vi "Execute.vi"(8 "error in (no error)":errorcluster, 10 "System In":refnum<class "abs_System.lvclass">, 11 "Node in":refnum<class "Parallel_Interleaved.lvclass">) -> (0 "error out":errorcluster, 1 "Status":T1, 2 "System Out":refnum<class "abs_System.lvclass">, 3 "Node out":refnum<class "Parallel_Interleaved.lvclass">)   [LabVIEW 2021, in "BT.lvlib" / "Parallel_Interleaved.lvclass"]
uses:
  Parallel_Interleaved/Parallel_Interleaved.lvclass
  C:/Users/Tim/Documents/GitHub/LV_Behaviour_Tree/Source/Support/abs_Composite/abs_Composite.lvclass
  C:/Users/Tim/Documents/GitHub/LV_Behaviour_Tree/Source/Support/abs_Parallel/abs_Parallel.lvclass
  abs_Node/Status.ctl
  abs_System/abs_System.lvclass
  Parallel_Interleaved/Parallel_Interleaved.lvclass/Parallel_Interleaved.ctl
  abs_Composite/abs_Composite.lvclass/abs_Composite.ctl
  abs_Composite/Properties/Read Index.vi
  abs_Composite/Properties/Read Num Nodes.vi
  abs_Composite/Properties/Write Index.vi
  Parallel_Interleaved/Properties/Read Always Repeat First Node.vi
  abs_Parallel.lvclass
  abs_Node/abs_Node.lvclass
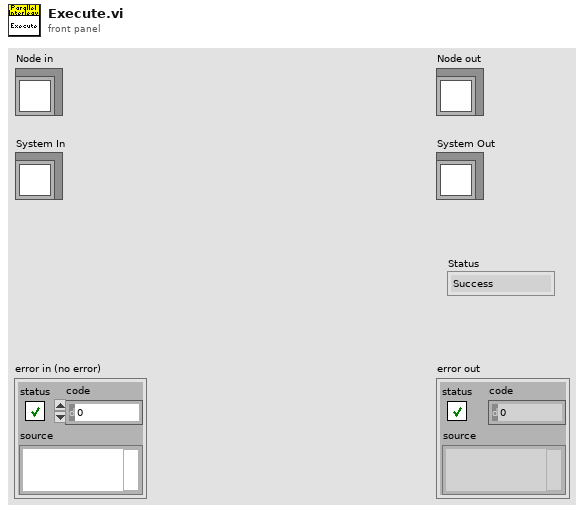
[diagram p1: front panel]
types:
  T1 = typedef "BT.lvlib/abs_Node.lvclass/Status.ctl" = enum16{"Success", "Failure", "Running"}
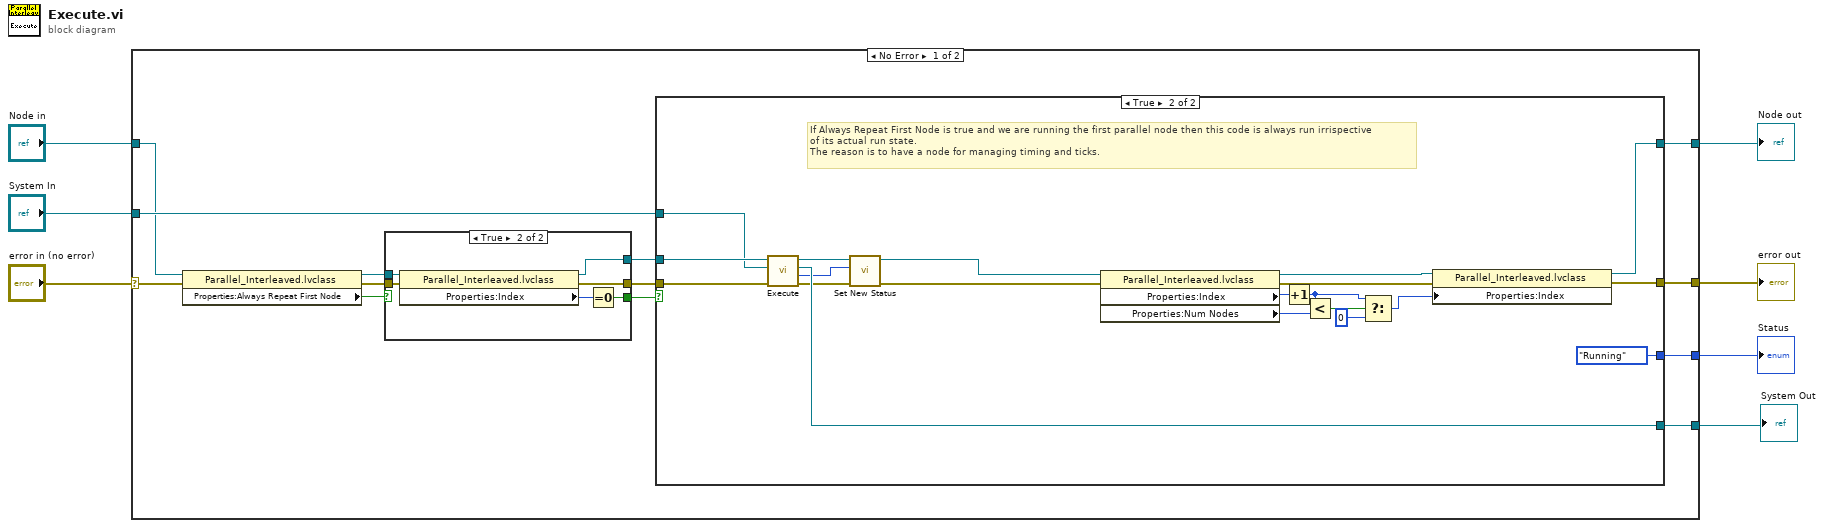
[diagram p0: block diagram]
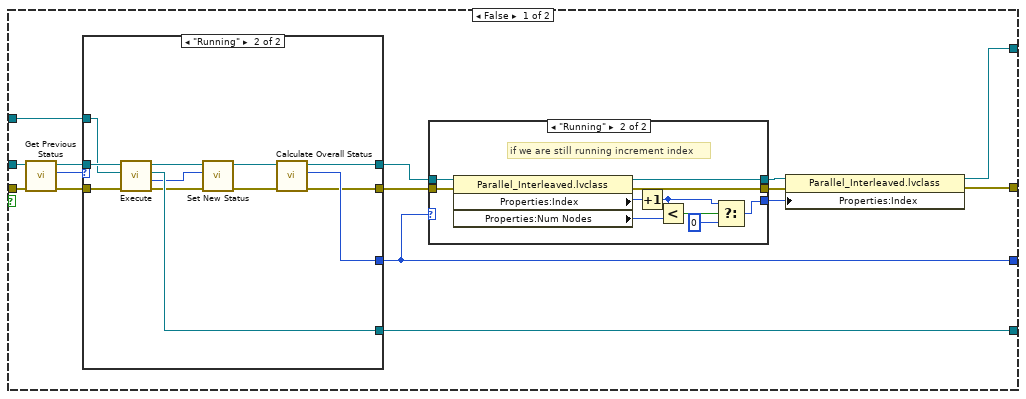
[diagram p2: hidden frame]
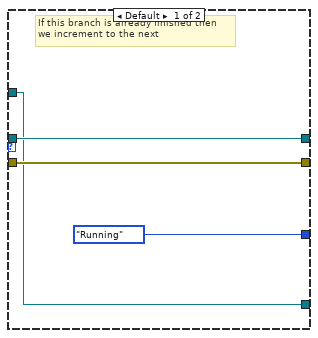
[diagram p3: hidden frame]
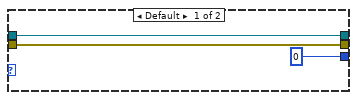
[diagram p4: hidden frame]
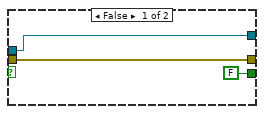
[diagram p5: hidden frame]
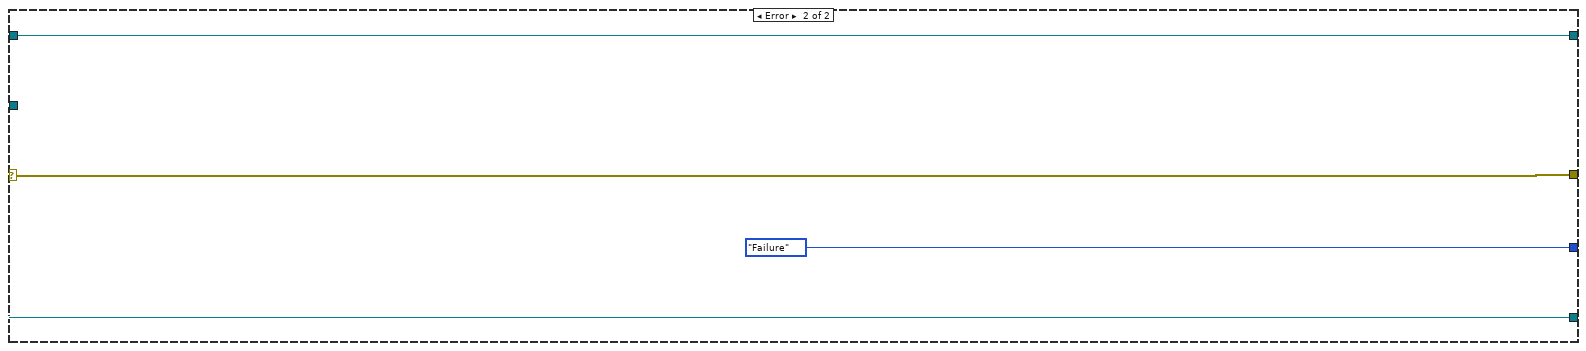
[diagram p6: hidden frame]
diagram:
  n1 = case shown="No Error" "error in (no error)" {
    selector: "error in (no error)" -> [w15 w96]
    tunnel: [w20 w95] -> w2
    tunnel: "System In" -> [w16 w95]
    tunnel: "Node in" -> [w14 w97]
    tunnel: [w19 w96] -> w4
    tunnel: [w18 w97] -> w1
    tunnel: [w17 Status."Failure" ("Status")] -> w3
    frame No Error {
      n2 = property class="Parallel_Interleaved.lvclass"(reference=w14, error in=w15) -> (reference out=w13:refnum<class "Parallel_Interleaved.lvclass">, error out=w12:errorcluster, "Properties:Always Repeat First Node"=w9:bool)
      n3 = case shown="True" w9 {
        tunnel: w13 -> [w87 w93]
        tunnel: w12 -> [w86 w92]
        tunnel: [w87 w91] -> w11
        tunnel: [w86 w90] -> w10
        tunnel: [FALSE w88] -> w8
        frame False {
        }
        frame True {
          n4 = property class="Parallel_Interleaved.lvclass"(reference=w93, error in=w92) -> (reference out=w91:refnum<class "Parallel_Interleaved.lvclass">, error out=w90:errorcluster, "Properties:Index"=w89:i32)
          n5 = Equal To 0?(x=w89) -> (x = 0?=w88:bool)
        }
      }
      n6 = case shown="True" w8 {
        tunnel: [w35 w84] -> w20
        tunnel: [w34 w83] -> w19
        tunnel: [w33 w82] -> w18
        tunnel: [w28 Status."Running" ("Overall Status")] -> w17
        tunnel: w16 -> [w23 w76]
        tunnel: w11 -> [w22 w77]
        tunnel: w10 -> [w21 w78]
        frame False {
          n7 = call "Get Previous Status.vi"("error in (no error)"=w21, "abs_Parallel in"=w22) -> ("error out"=w26:errorcluster, "Previous Status"=w24:T1, "abs_Parallel out"=w25:refnum<class "Parallel_Interleaved.lvclass">)  [unwired: 7 in]
          n8 = case shown="\"Running\"" w24 {
            tunnel: [w36 w51] -> w35
            tunnel: w23 -> [w36 w48]
            tunnel: [w39 w46] -> w32
            tunnel: [w38 w45] -> w29
            tunnel: [Status."Running" ("y") w47] -> w28
            tunnel: w25 -> [w39 w50]
            tunnel: w26 -> [w38 w49]
            frame Default {
              # "If this branch is already finished then \nwe increment to the next"
            }
            frame "Running" {
              n9 = call-parent "Execute.vi"("error in (no error)"=w49, "System In"=w48, "Node in"=w50) -> ("error out"=w43:errorcluster, "Status"=w42:T1, "System Out"=w51:refnum<class "abs_System.lvclass">, "Node out"=w44:refnum<class "Parallel_Interleaved.lvclass">)  [unwired: 5 in]
              n10 = call "Set New Status.vi"("error in (no error)"=w43, "Status"=w42, "abs_Parallel in"=w44) -> ("error out"=w40:errorcluster, "abs_Parallel out"=w41:refnum<class "Parallel_Interleaved.lvclass">)  [unwired: 7 in]
              n11 = call "Calculate Overall Status.vi"("error in (no error)"=w40, "abs_Parallel in"=w41) -> ("error out"=w45:errorcluster, "Overall Status"=w47:T1, "abs_Parallel out"=w46:refnum<class "Parallel_Interleaved.lvclass">)  [unwired: 7 in]
            }
          }
          n12 = case shown="\"Running\"" w28 {
            tunnel: w32 -> [w54 w62]
            tunnel: [w54 w61] -> w31
            tunnel: [0 ("f") w58] -> w30
            tunnel: w29 -> [w53 w56]
            tunnel: [w53 w55] -> w27
            frame Default {
            }
            frame "Running" {
              # "if we are still running increment index"
              n13 = property class="Parallel_Interleaved.lvclass"(reference=w62, error in=w56) -> (reference out=w61:refnum<class "Parallel_Interleaved.lvclass">, error out=w55:errorcluster, "Properties:Index"=w64:i32, "Properties:Num Nodes"=w63:i32)
              n14 = Increment(x=w64) -> (x+1=w59:i32)
              n15 = Less?(x=w59, y=w63) -> (x < y?=w60:bool)
              n16 = Select(t=w59, s=w60, f=0) -> (s? t:f=w58:i32)
            }
          }
          n17 = property class="Parallel_Interleaved.lvclass"(reference=w31, error in=w27, "Properties:Index"=w30) -> (reference out=w33:refnum<class "Parallel_Interleaved.lvclass">, error out=w34:errorcluster)
        }
        frame True {
          # "If Always Repeat First Node is true and we are running the first parallel node then this code is always run irrispective\nof its actual run state.\nThe reason is to have a node for managing timing and ticks."
          n18 = call-parent "Execute.vi"("error in (no error)"=w78, "System In"=w76, "Node in"=w77) -> ("error out"=w74:errorcluster, "Status"=w73:T1, "System Out"=w84:refnum<class "abs_System.lvclass">, "Node out"=w75:refnum<class "Parallel_Interleaved.lvclass">)  [unwired: 5 in]
          n19 = call "Set New Status.vi"("error in (no error)"=w74, "Status"=w73, "abs_Parallel in"=w75) -> ("error out"=w71:errorcluster, "abs_Parallel out"=w72:refnum<class "Parallel_Interleaved.lvclass">)  [unwired: 7 in]
          n20 = property class="Parallel_Interleaved.lvclass"(reference=w72, error in=w71) -> (reference out=w81:refnum<class "Parallel_Interleaved.lvclass">, error out=w79:errorcluster, "Properties:Index"=w70:i32, "Properties:Num Nodes"=w69:i32)
          n21 = Increment(x=w70) -> (x+1=w67:i32)
          n22 = Less?(x=w67, y=w69) -> (x < y?=w68:bool)
          n23 = Select(t=w67, s=w68, f=0) -> (s? t:f=w80:i32)
          n24 = property class="Parallel_Interleaved.lvclass"(reference=w81, error in=w79, "Properties:Index"=w80) -> (reference out=w82:refnum<class "Parallel_Interleaved.lvclass">, error out=w83:errorcluster)
        }
      }
    }
    frame Error {
    }
  }
  "error out" <- w4
  "Node out" <- w1
  "Status" <- w3
  "System Out" <- w2
